vi "(SubVI) Open a Glimpse to Write.vi"(3 "error in":errorcluster, 4 "index file (0,1,2,...)":i32, 5 "String Path Array":string[](array[string])) -> (0 "error out":errorcluster, 2 "Byte Stream File out":refnum<file>)   [LabVIEW 2014]
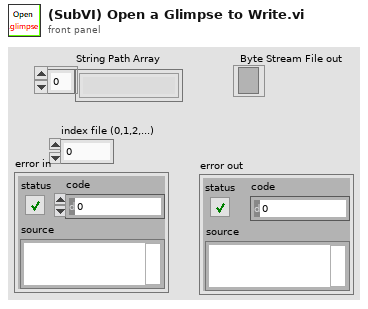
[diagram p1: front panel]
types:
  T1 = enum16{"open", "replace", "create", "open or create", "replace or create", "replace or create with confirmation"}
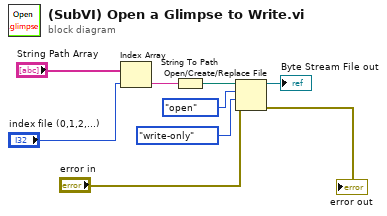
[diagram p0: block diagram]
diagram:
  n1 = Index Array(array="String Path Array", index="index file (0,1,2,...)") -> (element=w5:string)
  n2 = String To Path(string=w5) -> (path=w4:path)
  n3 = Open/Create/Replace File(file path (use dialog)=w4, error in="error in", operation (0:open)=T1."open", access (0:read/write)=enum16{"read/write", "read-only", "write-only"}."write-only") -> (refnum out=→"Byte Stream File out":refnum<file>, error out=→"error out":errorcluster)  [unwired: 2 in, 1 out]
